vi "Secure-Release Region.vi"(6 "Pickup_Test_Number":dbl, 7 "Action":enum16{"Secure", "Release"}(ring), 8 "error in (no error)":errorcluster, 10 "Control In":T1={"I-O.lvclass"=refnum, "Gantry"=refnum, "Dispenser"="COM1"}, 11 "Carrier Tray in":refnum<class "Assembly Tray.lvclass">) -> (0 "error out":errorcluster, 1 "Position":i32, 2 "Control Out":T1={"I-O.lvclass"=refnum, "Gantry"=refnum, "Dispenser"="COM1"}, 3 "Carrier Tray out":refnum<class "Assembly Tray.lvclass">)   [LabVIEW 2021, in "Assembly Tray.lvclass"]
uses:
  Assembly Tray.lvclass
  C:/Users/HEP/Documents/GitHub/Gantry/UCSB-Gantry-HEP-main/Classes/Workspace/Fixture.lvclass
  Controller/Controllers.ctl
  Controller/I-O/I-O.lvclass
  C:/Program Files (x86)/Aerotech/A3200/LabVIEW/2010/Bin/Aerotech.A3200.dll
  Program Files (x86)/Aerotech/A3200/LabVIEW/2010/Bin/Aerotech.A3200.dll
  Fixture.lvclass/Fixture.ctl
  Assembly Tray.lvclass/Assembly Tray.ctl
  Fixture.lvclass
  Controller/Controller.lvclass
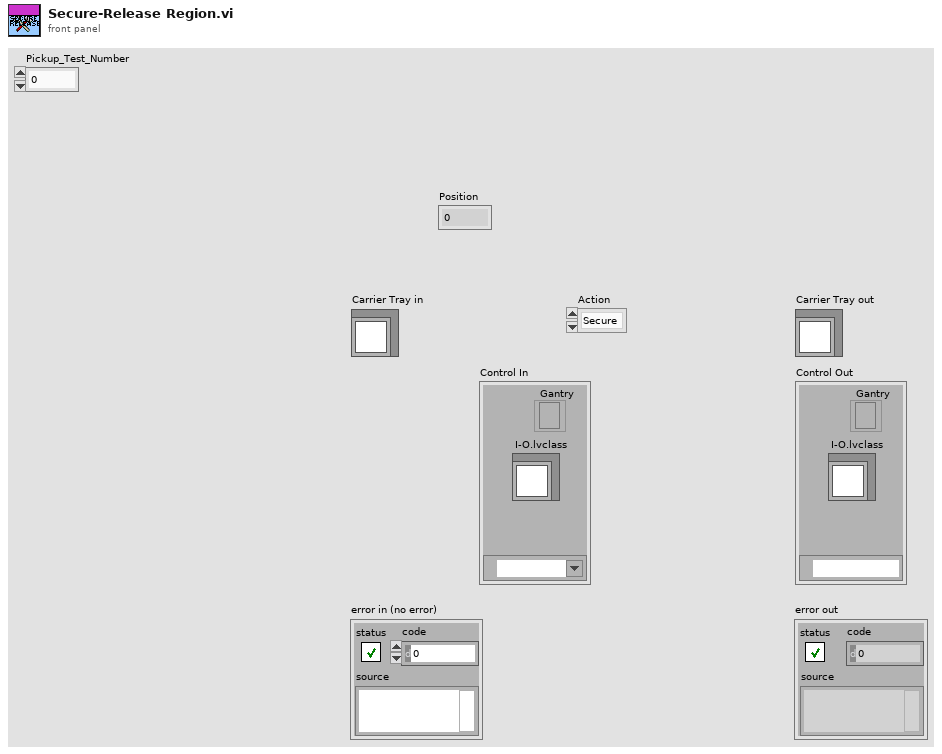
[diagram p1: front panel]
types:
  T1 = typedef "Controller.lvclass/Controllers.ctl" = cluster{"I-O.lvclass":refnum<class "I-O.lvclass">, "Gantry":refnum<k24>, "Dispenser":refnum<visa-resource-name>}
  T2 = typedef "I-O.lvclass/Pin Map.ctl" = cluster{"Region Valves":i32[], "Extra Valves":dbl[][][], "Tool Primary Valve":i32, "Tool Secondary Valve":i32, "Region Sensors":i32[], "Extra Sensors":dbl[][][], "Tool Primary Sensor":dbl, "Tool Secondary Sensor":dbl, "Compression Sensor":dbl, "5V":i32, "Dispenser Sensor":dbl, "Light Curtain":i32}
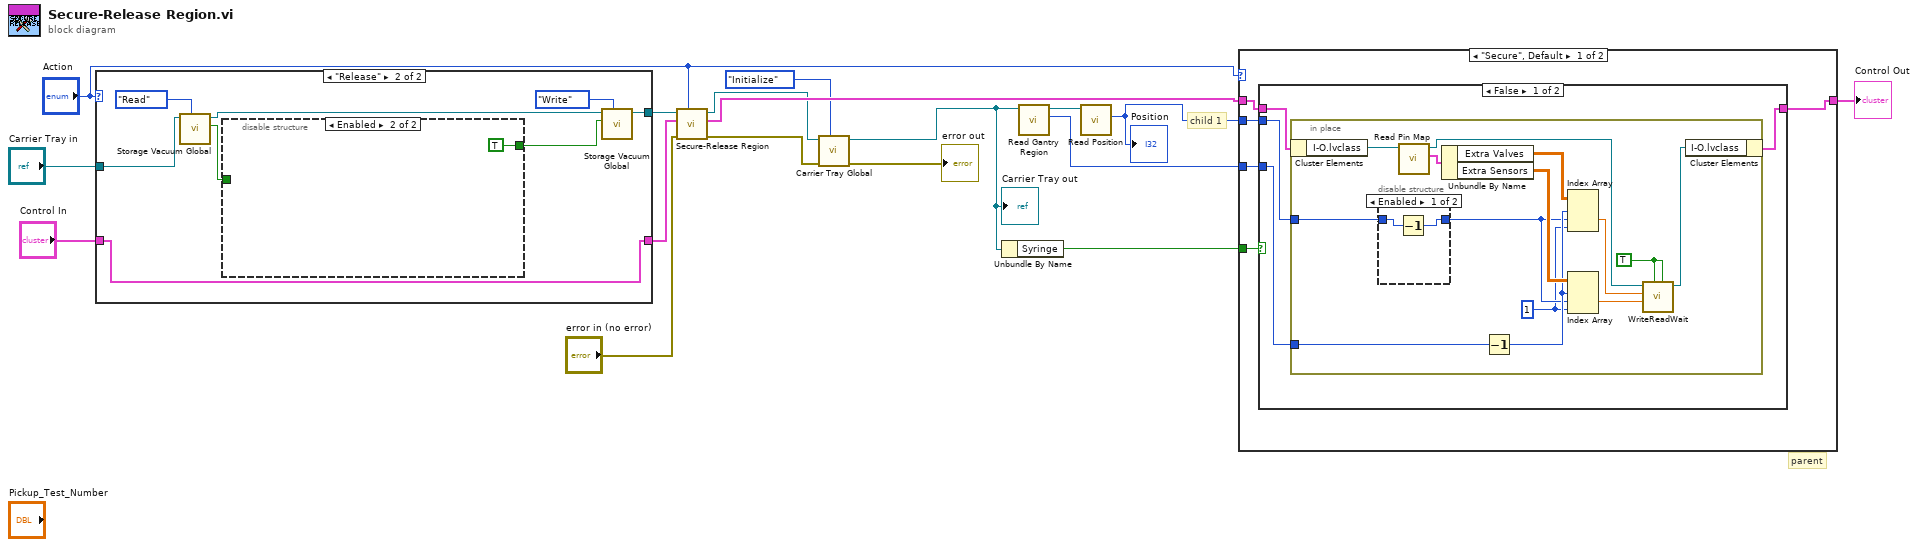
[diagram p0: block diagram]
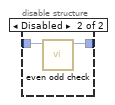
[diagram p2: hidden frame]
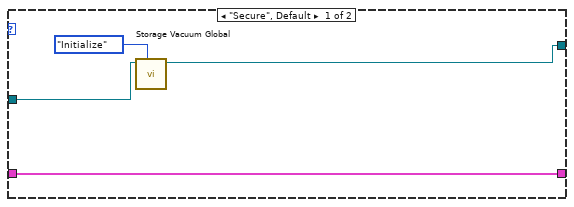
[diagram p5: hidden frame]
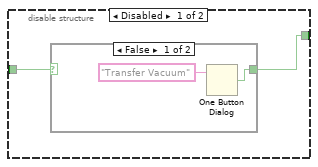
[diagram p6: hidden frame]
diagram:
  # "child 1"
  # "parent"
  n1 = case shown="\"Release\"" "Action" {
    tunnel: [w20 w25] -> w15
    tunnel: "Carrier Tray in" -> [w19 w24]
    tunnel: "Control In" -> [w18 w22]
    tunnel: [w18 w22] -> w1
    frame "Secure", Default {
      n2 = call "Storage Vacuum Global.vi"("Action"=enum16{"Initialize", "Read", "Write"}."Initialize", "Carrier Tray.lvclass"=w19) -> ("Carrier Tray.lvclass 2"=w20:refnum<class "Assembly Tray.lvclass">)  [unwired: 7 in, 2 out]
    }
    frame "Release" {
      n3 = call "Storage Vacuum Global.vi"("Action"=enum16{"Initialize", "Read", "Write"}."Read", "Carrier Tray.lvclass"=w24) -> ("Read"=w29:bool, "Carrier Tray.lvclass 2"=w26:refnum<class "Assembly Tray.lvclass">)  [unwired: 7 in, 1 out]
      n4 = disable-structure shown="Enabled" {
        disable-tunnel: w29 -> [w31 _]
        disable-tunnel: [w30 TRUE ("Write")] -> w23
        frame Disabled {
          n5 = case shown="False" w31 {
            selector: w31 -> [_ w34]
            tunnel: [w32 w34] -> w30
            frame False {
              n6 = One Button Dialog(message="Transfer Vacuum") -> (true=w32:bool)  [unwired: 1 in]
            }
            frame True {
            }
          }
        }
        frame Enabled {
        }
      }
      n7 = call "Storage Vacuum Global.vi"("Action"=enum16{"Initialize", "Read", "Write"}."Write", "Write"=w23, "Carrier Tray.lvclass"=w26) -> ("Carrier Tray.lvclass 2"=w25:refnum<class "Assembly Tray.lvclass">)  [unwired: 6 in, 2 out]
    }
  }
  n8 = call-parent "Secure-Release Region.vi"("Action"="Action", "error in (no error)"="error in (no error)", "Control In"=w1, "Fixture in"=w15) -> ("error out"=w5:errorcluster, "Control Out"=w13:T1, "Fixture out"=w8:refnum<class "Assembly Tray.lvclass">)  [unwired: 4 in, 1 out]
  n9 = call "Carrier Tray Global.vi"("Action"=enum16{"Initialize", "Read", "Write"}."Initialize", "error in (no error)"=w5, "Carrier Tray.lvclass"=w8) -> ("error out"=→"error out":errorcluster, "Carrier Tray.lvclass 2"=w7:refnum<class "Assembly Tray.lvclass">)  [unwired: 6 in, 1 out]
  "Carrier Tray out" <- w7
  n10 = Unbundle By Name(w7) -> ("Syringe"=w14:bool)
  n11 = call "Read Gantry Region.vi"("Fixture in"=w7) -> ("Gantry Region"=w11:i32, "Fixture out"=w12:refnum<class "Assembly Tray.lvclass">)  [unwired: 8 in, 1 out]
  n12 = call "Read Position.vi"("Fixture in"=w12) -> ("Position"=w3:i32)  [unwired: 8 in, 2 out]
  "Position" <- w3
  n13 = case shown="\"Secure\", Default" "Action" {
    tunnel: w14 -> [w40 _]
    tunnel: w13 -> [w39 w64]
    tunnel: w11 -> [w38 _]
    tunnel: w3 -> [w37 _]
    tunnel: [w36 w64] -> w10
    frame "Secure", Default {
      n14 = case shown="False" w40 {
        tunnel: w39 -> [w44 w63]
        tunnel: w38 -> [w43 _]
        tunnel: w37 -> [w42 _]
        tunnel: [w41 w63] -> w36
        frame False {
          n15 = in-place {
            in-place-border: w43 -> [w52]
            in-place-border: w42 -> [w50]
            w48 = 1
            w54 = TRUE
            n16 = in-place-cluster #1(w44) -> ("I-O.lvclass"=w58:refnum<class "I-O.lvclass">)
            n17 = disable-structure shown="Enabled" {
              disable-tunnel: w50 -> [w60 w62]
              disable-tunnel: [w59 w61] -> w49
              frame Enabled {
                n18 = Decrement(x=w60) -> (x-1=w59:i32)
              }
              frame Disabled {
                n19 = call "even odd check.vi"("position"=w62) -> ("index"=w61:i32)  [unwired: 10 in]
              }
            }
            n20 = call-dynamic "Read Pin Map.vi"("I-O in"=w58) -> ("Pin Map 2"=w57:T2, "I-O out"=w55:refnum<class "I-O.lvclass">)  [unwired: 8 in, 1 out]
            n21 = Unbundle By Name(w57) -> ("Extra Valves"=w45:dbl[][][], "Extra Sensors"=w56:dbl[][][])
            n22 = Decrement(x=w52) -> (x-1=w51:i32)
            n23 = Index Array(array=w45, index (dim 0)=w51, index (dim 1)=w49, index (dim 2)=w48) -> (element=w47:dbl)
            n24 = Index Array(array=w56, index (dim 0)=w51, index (dim 1)=w49, index (dim 2)=w48) -> (element=w46:dbl)
            n25 = call "WriteReadWait.vi"("Read Value"=w54, "Write Value"=w54, "Read"=w46, "Write"=w47, "I-O in"=w55) -> ("I-O out"=w53:refnum<class "I-O.lvclass">)  [unwired: 5 in, 1 out]
            n26 = in-place-cluster #1("I-O.lvclass"=w53) -> (w41:T1)
          }
        }
        frame True {
        }
      }
    }
    frame "Release" {
    }
  }
  "Control Out" <- w10
